vi "ExternalVIDefaultCheckUpdate.vi"(3 "OP":enum16{"Get", "Update", "Init"}(ring), 4 "last mod":timestamp, 5 "VIName":string="VIName") -> (0 "VINameFind?":bool, 1 "NeedUpdate?":bool=TRUE)   [LabVIEW 2020]
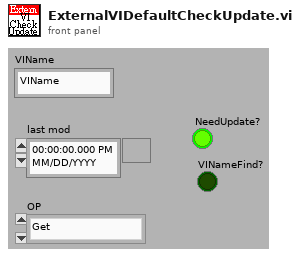
[diagram p1: front panel]
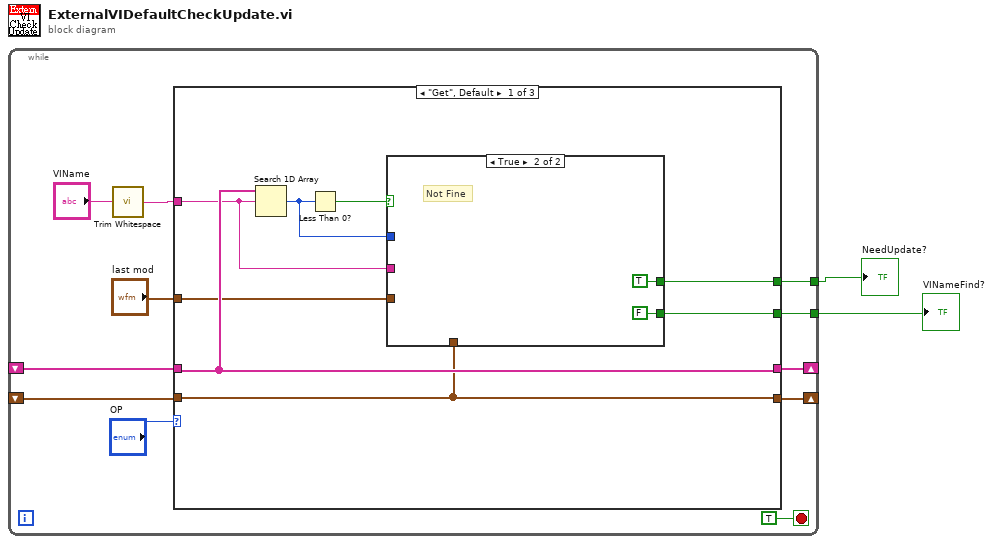
[diagram p0: block diagram]
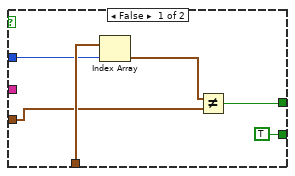
[diagram p2: hidden frame]
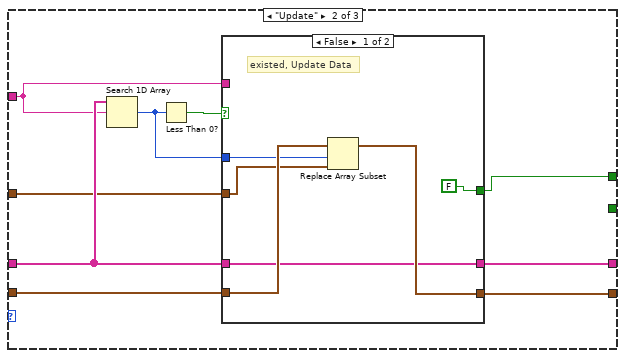
[diagram p3: hidden frame]
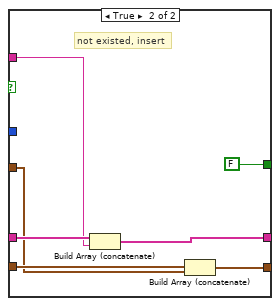
[diagram p4: hidden frame]
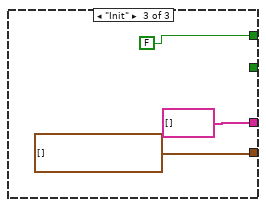
[diagram p5: hidden frame]
diagram:
  n1 = while {
    shift-right: [w11] -> _
    shift-left: _ -> [w10]
    shift-right: [w7] -> _
    shift-left: _ -> [w6]
    tunnel: [w5] -> w2
    tunnel: [w4] -> w1
    stop <- TRUE stop-if-true
    n2 = call <vilib>:"Trim Whitespace.vi"("string"="VIName") -> ("trimmed string"=w8:string)  [unwired: 1 in]
    n3 = case shown="\"Get\", Default" "OP" {
      tunnel: [w21 w34 string[] [] ("DeviceList")] -> w11
      tunnel: w10 -> [w21 w35 _]
      tunnel: w8 -> [w16 w33 _]
      tunnel: w6 -> [w18 w37 _]
      tunnel: [w18 w32 timestamp[] []] -> w7
      tunnel: [w17 w31 FALSE] -> w5
      tunnel: [w15 _ _] -> w4
      tunnel: "last mod" -> [w14 w30 _]
      frame "Get", Default {
        n4 = Search 1D Array(1D array=w21, element=w16) -> (index of element=w19:i32)  [unwired: 1 in]
        n5 = Less Than 0?(x=w19) -> (x < 0?=w20:bool)
        n6 = case shown="True" w20 {
          tunnel: w18 -> [w27 _]
          tunnel: w19 -> [w26 _]
          tunnel: [w24 TRUE] -> w17
          tunnel: w16 -> [_ _]
          tunnel: [TRUE ("BusyStateIn") FALSE ("BusyStateIn")] -> w15
          tunnel: w14 -> [w22 _]
          frame False {
            n7 = Index Array(array=w27, index=w26) -> (element=w23:timestamp)
            n8 = Not Equal?(x=w23, y=w22) -> (x != y?=w24:bool)
          }
          frame True {
            # "Not Fine"
          }
        }
      }
      frame "Update" {
        n9 = Search 1D Array(1D array=w35, element=w33) -> (index of element=w36:i32)  [unwired: 1 in]
        n10 = Less Than 0?(x=w36) -> (x < 0?=w38:bool)
        n11 = case shown="False" w38 {
          tunnel: w37 -> [w44 w48]
          tunnel: w36 -> [w43 _]
          tunnel: w30 -> [w40 w46]
          tunnel: [w42 w47] -> w32
          tunnel: w35 -> [w41 w51]
          tunnel: [w41 w49] -> w34
          tunnel: w33 -> [_ w50]
          tunnel: [FALSE FALSE] -> w31
          frame False {
            # "existed, Update Data"
            n12 = Replace Array Subset(array=w44, new element=w40, index=w43) -> (w42:timestamp[])
          }
          frame True {
            # "not existed, insert"
            n13 = Build Array (concatenate)(w51, w50) -> (w49:string[])
            n14 = Build Array (concatenate)(w48, w46) -> (w47:timestamp[])
          }
        }
      }
      frame "Init" {
      }
    }
  }
  "NeedUpdate?" <- w2
  "VINameFind?" <- w1
